vi "Save Images.vi"(6 "Time Stamp":timestamp, 8 "error in (no error)":errorcluster, 9 "Left Image":T1, 10 "Right Image":T1, 11 "Save File Path":path) -> (0 "error out":errorcluster)   [LabVIEW 2012]
uses:
  <vilib>/vision/Image Controls.llb/IMAQ Image.ctl
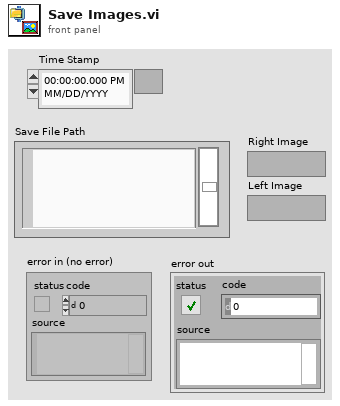
[diagram p1: front panel]
types:
  T1 = typedef "IMAQ Image.ctl" = refnum<image>
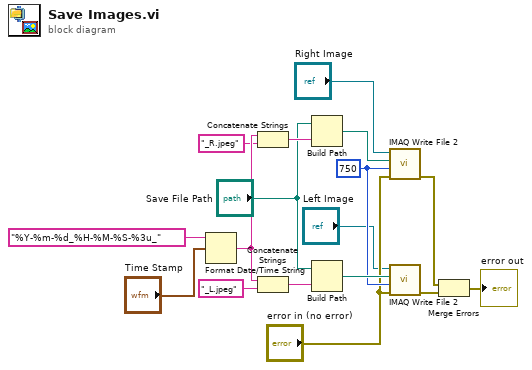
[diagram p0: block diagram]
diagram:
  w6 = u32 750 ("Image Quality")
  n1 = Format Date/Time String(time format string (%c)="%Y-%m-%d_%H-%M-%S-%3u_", seconds (now)="Time Stamp") -> (date/time string=w14:string)  [unwired: 1 in]
  n2 = Concatenate Strings(w14, "_R.jpeg") -> (w11:string)
  n3 = Concatenate Strings(w14, "_L.jpeg") -> (w7:string)
  n4 = Build Path(base path="Save File Path", name or relative path=w11) -> (appended path=w10:path)
  n5 = Build Path(base path="Save File Path", name or relative path=w7) -> (appended path=w9:path)
  n6 = call-poly "IMAQ Write File 2"("error in (no error)"="error in (no error)", "Image Quality"=w6, "File Path"=w10, "Image"="Right Image") -> ("error out"=w16:errorcluster)  [unwired: 6 in, 1 out]
  n7 = call-poly "IMAQ Write File 2"("error in (no error)"="error in (no error)", "Image Quality"=w6, "File Path"=w9, "Image"="Left Image") -> ("error out"=w15:errorcluster)  [unwired: 6 in, 1 out]
  n8 = Merge Errors(w16, w15) -> (→"error out":errorcluster)
